vi "FFT_CC.vi"(8 "error in (no error)":errorcluster, 10 "Roy":T1, 11 "Rob":T1) -> (0 "error out":errorcluster, 3 "Phase correlation out":T1)   [LabVIEW 2012]
uses:
  <vilib>/vision/Image Controls.llb/IMAQ Image.ctl
  <vilib>/vision/NI_Vision_Development_Module.lvlib
panel:
  out "Phase correlation monitor":T1(plugin-control)
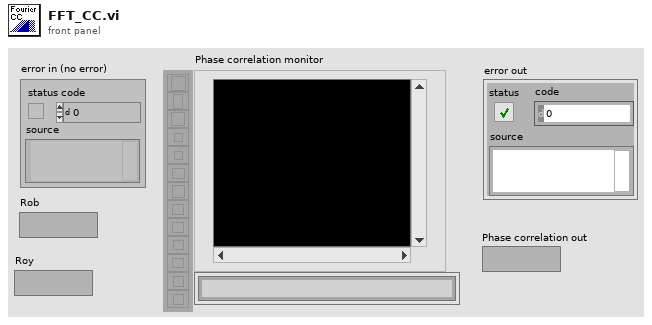
[diagram p1: front panel]
types:
  T1 = typedef "IMAQ Image.ctl" = refnum<image>
  T2 = enum32{"Real", "Imaginary", "Magnitude", "Phase"}
  T3 = typedef "Image Type" = u32
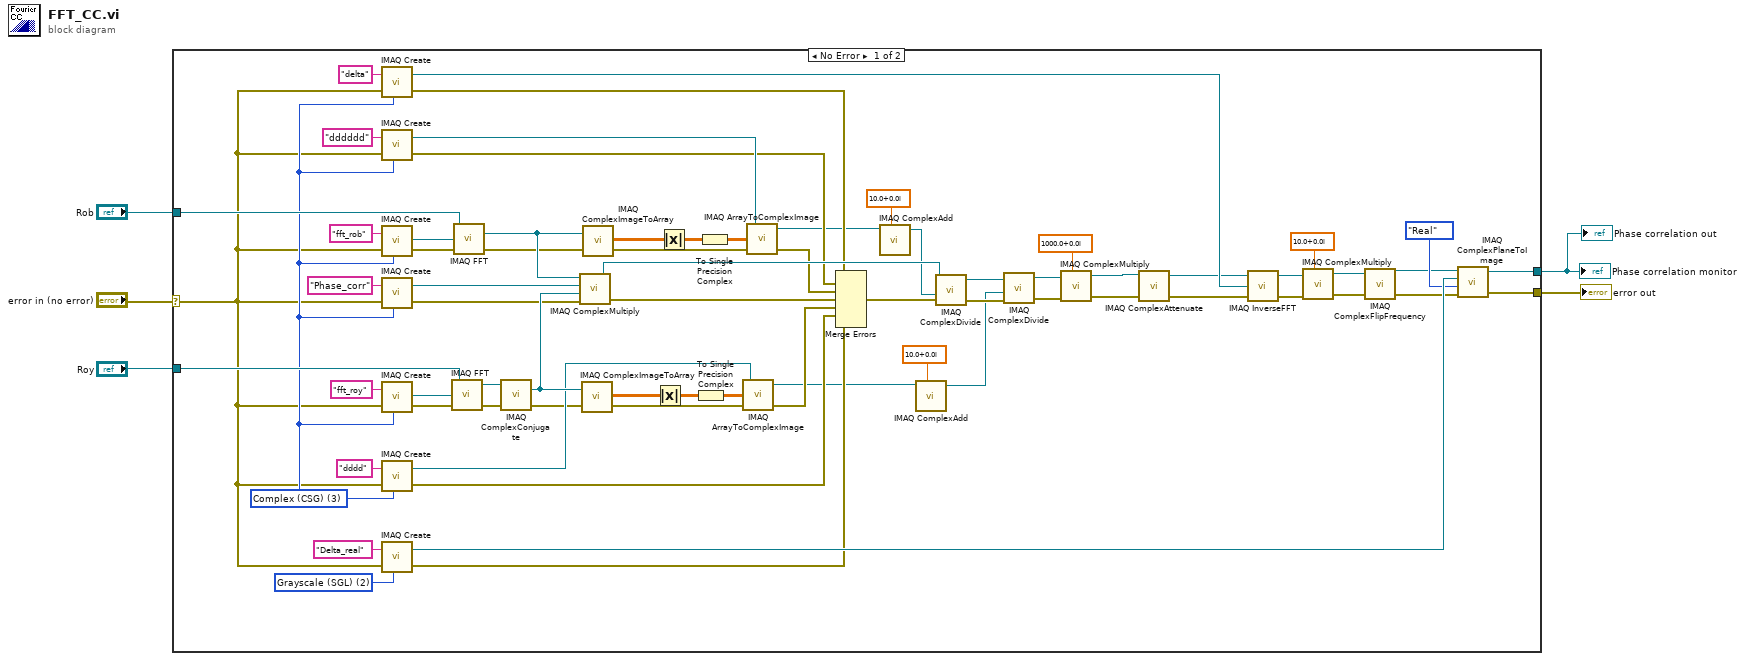
[diagram p0: block diagram]
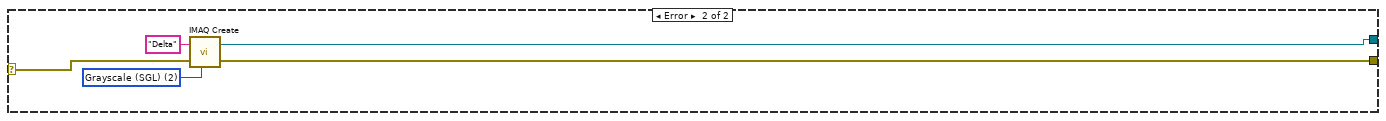
[diagram p2: hidden frame]
diagram:
  n1 = case shown="No Error" "error in (no error)" {
    selector: "error in (no error)" -> [w20 w78]
    tunnel: "Rob" -> [w43 _]
    tunnel: "Roy" -> [w42 _]
    tunnel: [w19 w76] -> w2
    tunnel: [w18 w77] -> w1
    frame No Error {
      w46 = T3 2 items=["Grayscale (U8)", "Grayscale (I16)", "Grayscale (SGL)", "Complex (CSG)", "RGB (U32)", "HSL (U32)", "RGB (U64)", "Grayscale (U16)"] ("Image Type")
      w31 = T3 3 items=["Grayscale (U8)", "Grayscale (I16)", "Grayscale (SGL)", "Complex (CSG)", "RGB (U32)", "HSL (U32)", "RGB (U64)", "Grayscale (U16)"] ("Image Type")
      n2 = call "IMAQ Create"("Image Name"="delta", "Image Type"=w31, "error in (no error)"=w20) -> ("New Image"=w59:T1, "error out"=w28:errorcluster)  [unwired: 2 in]
      n3 = call "IMAQ Create"("Image Name"="dddddd", "Image Type"=w31, "error in (no error)"=w20) -> ("New Image"=w51:T1, "error out"=w27:errorcluster)  [unwired: 2 in]
      n4 = call "IMAQ Create"("Image Name"="fft_rob", "Image Type"=w31, "error in (no error)"=w20) -> ("New Image"=w73:T1, "error out"=w41:errorcluster)  [unwired: 2 in]
      n5 = call "IMAQ Create"("Image Name"="Phase_corr", "Image Type"=w31, "error in (no error)"=w20) -> ("New Image"=w69:T1, "error out"=w37:errorcluster)  [unwired: 2 in]
      n6 = call "IMAQ Create"("Image Name"="fft_roy", "Image Type"=w31, "error in (no error)"=w20) -> ("New Image"=w72:T1, "error out"=w40:errorcluster)  [unwired: 2 in]
      n7 = call "IMAQ Create"("Image Name"="dddd", "Image Type"=w31, "error in (no error)"=w20) -> ("New Image"=w50:T1, "error out"=w23:errorcluster)  [unwired: 2 in]
      n8 = call "IMAQ Create"("Image Name"="Delta_real", "Image Type"=w46, "error in (no error)"=w20) -> ("New Image"=w47:T1, "error out"=w22:errorcluster)  [unwired: 2 in]
      n9 = call "IMAQ FFT"("error in (no error)"=w40, "Image Dst"=w72, "Image Src"=w42) -> ("error out"=w39:errorcluster, "Image Dst Out"=w71:T1)  [unwired: 1 in]
      n10 = call "IMAQ FFT"("error in (no error)"=w41, "Image Dst"=w73, "Image Src"=w43) -> ("error out"=w36:errorcluster, "Image Dst Out"=w58:T1)  [unwired: 1 in]
      n11 = call "IMAQ ComplexConjugate"("error in (no error)"=w39, "Image Src"=w71) -> ("error out"=w38:errorcluster, "Image Dst Out"=w57:T1)  [unwired: 2 in]
      n12 = call "IMAQ ComplexMultiply"("Image Src A"=w58, "Image Dst"=w69, "Image Src B"=w57, "error in (no error)"=w37) -> ("Image Dst Out"=w62:T1, "error out"=w25:errorcluster)  [unwired: 3 in]
      n13 = call "IMAQ ComplexImageToArray"("Image"=w57, "error in (no error)"=w38) -> ("Image Pixels (Complex)"=w65:csg[][], "error out"=w35:errorcluster)  [unwired: 3 in]
      n14 = call "IMAQ ComplexImageToArray"("Image"=w58, "error in (no error)"=w36) -> ("Image Pixels (Complex)"=w68:csg[][], "error out"=w34:errorcluster)  [unwired: 3 in]
      n15 = Absolute Value(x=w65) -> (abs(x)=w64:sgl[][])
      n16 = Absolute Value(x=w68) -> (abs(x)=w67:sgl[][])
      n17 = To Single Precision Complex(1:w64) -> (0:w63:csg[][])
      n18 = To Single Precision Complex(1:w67) -> (0:w66:csg[][])
      n19 = call "IMAQ ArrayToComplexImage"("error in (no error)"=w35, "Image Pixels (Complex)"=w63, "Image"=w50) -> ("error out"=w24:errorcluster, "Image Out"=w11:T1)  [unwired: 1 in]
      n20 = call "IMAQ ArrayToComplexImage"("error in (no error)"=w34, "Image Pixels (Complex)"=w66, "Image"=w51) -> ("error out"=w26:errorcluster, "Image Out"=w7:T1)  [unwired: 1 in]
      n21 = Merge Errors(w28, w27, w26, w25, w24, w23, w22) -> (w21:errorcluster)
      n22 = call "IMAQ ComplexAdd"("Image Src A"=w7, "Constant"=csg 10.0+0.0i) -> ("Image Dst Out"=w6:T1)  [unwired: 5 in, 1 out]
      n23 = call "IMAQ ComplexAdd"("Image Src A"=w11, "Constant"=csg 10.0+0.0i) -> ("Image Dst Out"=w10:T1)  [unwired: 5 in, 1 out]
      n24 = call "IMAQ ComplexDivide"("Image Src A"=w62, "Image Src B"=w6, "error in (no error)"=w21) -> ("Image Dst Out"=w61:T1, "error out"=w33:errorcluster)  [unwired: 4 in]
      n25 = call "IMAQ ComplexDivide"("Image Src A"=w61, "Image Src B"=w10, "error in (no error)"=w33) -> ("Image Dst Out"=w56:T1, "error out"=w32:errorcluster)  [unwired: 4 in]
      n26 = call "IMAQ ComplexMultiply"("Image Src A"=w56, "Constant"=csg 1000.0+0.0i, "error in (no error)"=w32) -> ("Image Dst Out"=w17:T1, "error out"=w15:errorcluster)  [unwired: 4 in]
      n27 = call "IMAQ ComplexAttenuate"("error in (no error)"=w15, "Image Src"=w17) -> ("error out"=w14:errorcluster, "Image Dst Out"=w16:T1)  [unwired: 3 in]
      n28 = call "IMAQ InverseFFT"("error in (no error)"=w14, "Image Dst"=w59, "Image Src"=w16) -> ("error out"=w30:errorcluster, "Image Dst Out"=w54:T1)  [unwired: 1 in]
      n29 = call "IMAQ ComplexMultiply"("Image Src A"=w54, "Constant"=csg 10.0+0.0i, "error in (no error)"=w30) -> ("Image Dst Out"=w13:T1, "error out"=w12:errorcluster)  [unwired: 4 in]
      n30 = call "IMAQ ComplexFlipFrequency"("error in (no error)"=w12, "Image Src"=w13) -> ("error out"=w29:errorcluster, "Image Dst Out"=w44:T1)  [unwired: 2 in]
      n31 = call "IMAQ ComplexPlaneToImage"("error in (no error)"=w29, "Plane"=T2."Real", "Image Dst"=w47, "Image Src"=w44) -> ("error out"=w18:errorcluster, "Image Dst Out"=w19:T1)  [unwired: 1 in]
    }
    frame Error {
      w79 = T3 2 items=["Grayscale (U8)", "Grayscale (I16)", "Grayscale (SGL)", "Complex (CSG)", "RGB (U32)", "HSL (U32)", "RGB (U64)", "Grayscale (U16)"] ("Image Type")
      n32 = call "IMAQ Create"("Image Name"="Delta", "Image Type"=w79, "error in (no error)"=w78) -> ("New Image"=w76:T1, "error out"=w77:errorcluster)  [unwired: 2 in]
    }
  }
  "Phase correlation monitor" <- w2
  "error out" <- w1
  "Phase correlation out" <- w2
